vi "Initiate Sweep.vi"(8 "error in":errorcluster, 9 "Channel (Channel A)":T1, 10 "Node In":string, 11 "VISA resource name":refnum<visa-resource-name>) -> (0 "error out":errorcluster, 2 "Node Out":string, 3 "VISA resource name out":refnum<visa-resource-name>, 4 "Command String":string)   [LabVIEW 2013, in "Keithley 2600 Series.lvlib"]
doc: "This VI initiates a sweep. It causes the SMU to clear the four trigger model event detectors and enter its trigger model state machine.\n\n<b>Remarks:</b>\nTo perform source actions during the sweep, it is necessary to call one of the sweep source configuration functions (smuX.trigger.source.linearX, smuX.trigger.source.listX, or smuX.trigger.source.logX) prior to calling this function. To perform measure actions during the sweep it is necessary to configure the measurement event prior to calling this function.\n\nThis VI initiates an overlapped operation.\n\n<b>Functions and Attributes Used</b>\nsmuX.trigger.initiate()"
uses:
  Keithley 2600 Series.lvlib
  Private/GlobalVariables.vi
  Channel.ctl
panel:
  # "(c) 2008 Keithley Instruments, Inc.  ALL RIGHTS RESERVED."
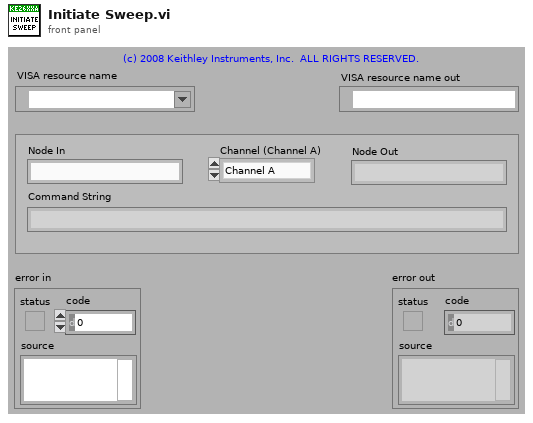
[diagram p1: front panel]
types:
  T1 = typedef "Keithley 2600 Series.lvlib/Channel.ctl" = enum32{"Channel A", "Channel B"}
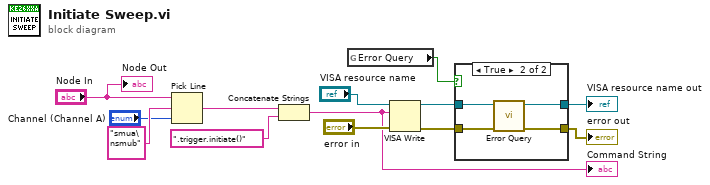
[diagram p0: block diagram]
diagram:
  n1 = Pick Line(string ("")="Node In", multi-line string="smua\nsmub", line index="Channel (Channel A)") -> (output string=w11:string)
  n2 = Concatenate Strings(w11, ".trigger.initiate()" ("string")) -> (w1:string)
  "Command String" <- w1
  n3 = global read "GlobalVariables.vi" "Error Query"() -> (w6:bool)
  n4 = VISA Write(VISA resource name="VISA resource name", write buffer=w1, error in (no error)="error in") -> (VISA resource name out=w5:refnum<visa-resource-name>, error out=w4:errorcluster)  [unwired: 1 out]
  n5 = case shown="True" w6 {
    tunnel: w5 -> [w15 w19]
    tunnel: w4 -> [w14 w18]
    tunnel: [w15 w17] -> w3
    tunnel: [w14 w16] -> w2
    frame False {
    }
    frame True {
      n6 = call "Error Query.vi"("error in (no error)"=w18, "VISA resource name"=w19) -> ("error out"=w16:errorcluster, "VISA resource name out"=w17:refnum<visa-resource-name>)  [unwired: 8 out]
    }
  }
  "VISA resource name out" <- w3
  "error out" <- w2
  "Node Out" <- "Node In"
